vi "AnalogTriggers.vi"(1 "Limits":T5, 2 "Sources":T4, 3 "DutyCycles":T1, 4 "AnalogInputs":u16[](array[numeric])=[0, 0, 0, 0, 0, 0, 0, 0]) -> (0 "Outputs":T2)   [LabVIEW 2019]
uses:
  Controls/AnalogTrigger_Limits.ctl
  Controls/AnalogTrigger_Sources.ctl
  Controls/AnalogTrigger_Outputs.ctl
  Helpers/AnalogTriggerOutput.ctl
  Controls/DutyCycle_Outputs.ctl
  <vilib>/rvi/Emulation/niFpgaSctlEmulationGetInTimedLoop.vi
  <vilib>/rvi/Emulation/niFpgaProcessEmulError.vi
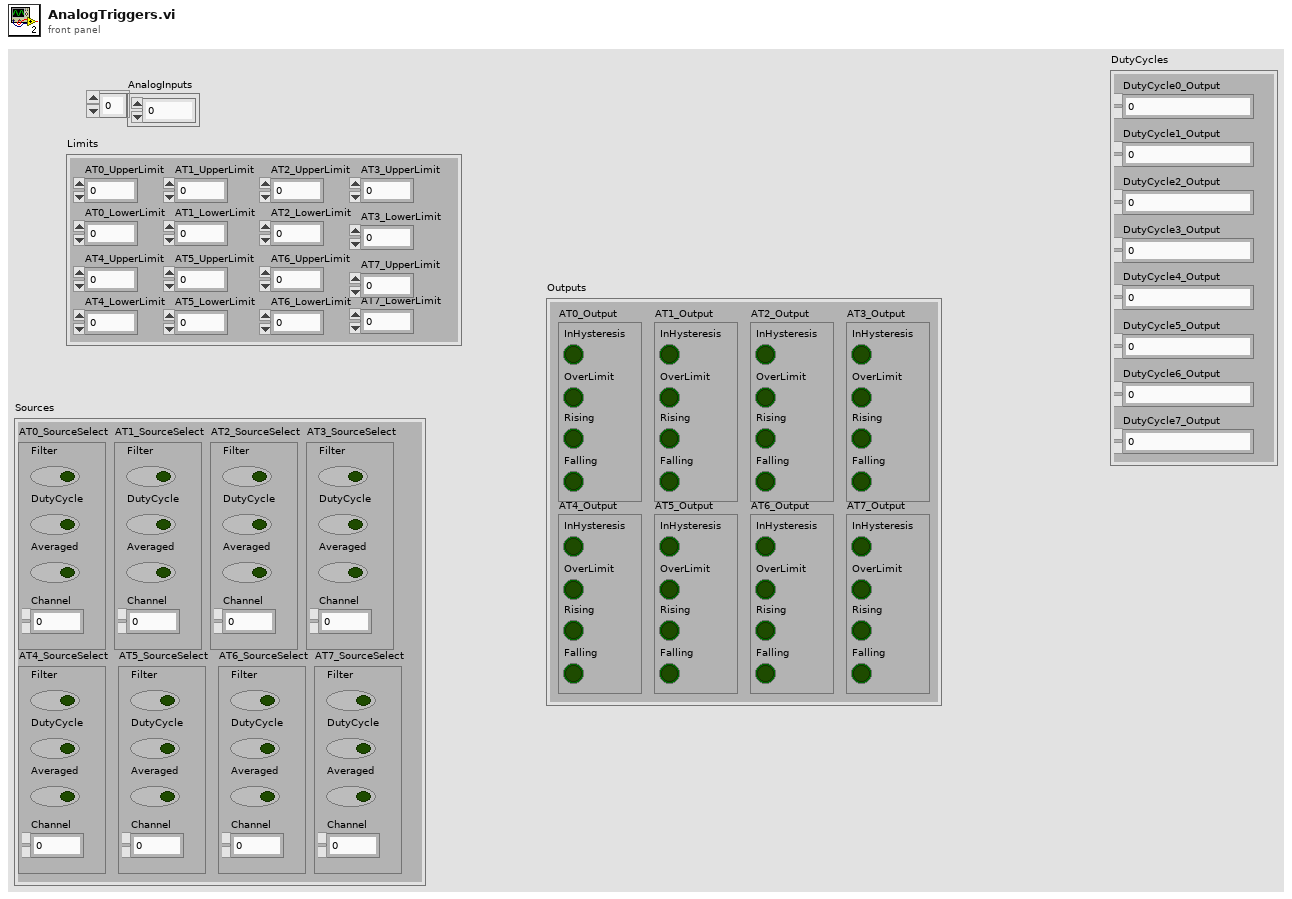
[diagram p1: front panel]
types:
  T1 = typedef "DutyCycle_Outputs.ctl" = cluster{"DutyCycle0_Output":fxp<+,31,31>, "DutyCycle1_Output":fxp<+,31,31>, "DutyCycle2_Output":fxp<+,31,31>, "DutyCycle3_Output":fxp<+,31,31>, "DutyCycle4_Output":fxp<+,31,31>, "DutyCycle5_Output":fxp<+,31,31>, "DutyCycle6_Output":fxp<+,31,31>, "DutyCycle7_Output":fxp<+,31,31>}
  T2 = typedef "AnalogTrigger_Outputs.ctl" = cluster{"AT0_Output":T3, "AT1_Output":T3, "AT2_Output":T3, "AT3_Output":T3, "AT4_Output":T3, "AT5_Output":T3, "AT6_Output":T3, "AT7_Output":T3}
  T3 = typedef "AnalogTriggerOutput.ctl" = cluster{"InHysteresis":bool, "OverLimit":bool, "Rising":bool, "Falling":bool}
  T4 = typedef "AnalogTrigger_Sources.ctl" = cluster{"AT0_SourceSelect":cluster{"Filter":bool, "DutyCycle":bool, "Averaged":bool, "Channel":fxp<+,3,3>}, "AT1_SourceSelect":cluster{"Filter":bool, "DutyCycle":bool, "Averaged":bool, "Channel":fxp<+,3,3>}, "AT2_SourceSelect":cluster{"Filter":bool, "DutyCycle":bool, "Averaged":bool, "Channel":fxp<+,3,3>}, "AT3_SourceSelect":cluster{"Filter":bool, "DutyCycle":bool, "Averaged":bool, "Channel":fxp<+,3,3>}, "AT4_SourceSelect":cluster{"Filter":bool, "DutyCycle":bool, "Averaged":bool, "Channel":fxp<+,3,3>}, "AT5_SourceSelect":cluster{"Filter":bool, "DutyCycle":bool, "Averaged":bool, "Channel":fxp<+,3,3>}, "AT6_SourceSelect":cluster{"Filter":bool, "DutyCycle":bool, "Averaged":bool, "Channel":fxp<+,3,3>}, "AT7_SourceSelect":cluster{"Filter":bool, "DutyCycle":bool, "Averaged":bool, "Channel":fxp<+,3,3>}}
  T5 = typedef "AnalogTrigger_Limits.ctl" = cluster{"AT0_LowerLimit":u32, "AT0_UpperLimit":u32, "AT1_LowerLimit":u32, "AT1_UpperLimit":u32, "AT2_LowerLimit":u32, "AT2_UpperLimit":u32, "AT3_LowerLimit":u32, "AT3_UpperLimit":u32, "AT4_LowerLimit":u32, "AT4_UpperLimit":u32, "AT5_LowerLimit":u32, "AT5_UpperLimit":u32, "AT6_LowerLimit":u32, "AT6_UpperLimit":u32, "AT7_LowerLimit":u32, "AT7_UpperLimit":u32}
  T6 = cluster{"Filter":bool, "DutyCycle":bool, "Averaged":bool, "Channel":fxp<+,3,3>}
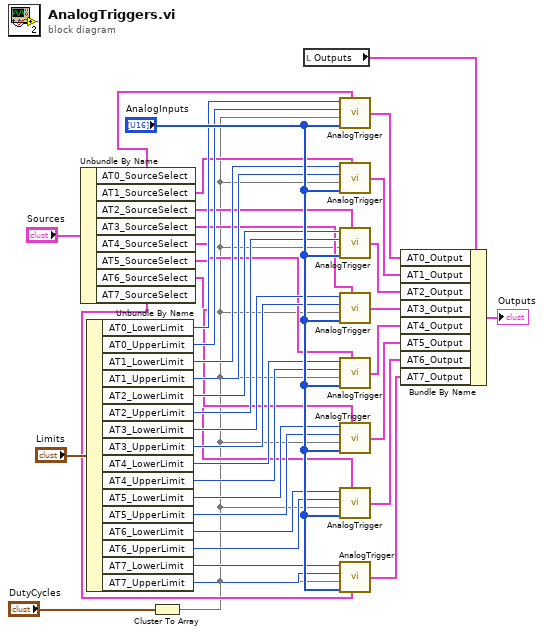
[diagram p0: block diagram]
diagram:
  n1 = Unbundle By Name("Sources") -> ("AT0_SourceSelect"=w20:T6, "AT1_SourceSelect"=w19:T6, "AT2_SourceSelect"=w18:T6, "AT3_SourceSelect"=w17:T6, "AT4_SourceSelect"=w16:T6, "AT5_SourceSelect"=w15:T6, "AT6_SourceSelect"=w14:T6, "AT7_SourceSelect"=w13:T6)
  n2 = Unbundle By Name("Limits") -> ("AT0_LowerLimit"=w37:u32, "AT0_UpperLimit"=w36:u32, "AT1_LowerLimit"=w35:u32, "AT1_UpperLimit"=w34:u32, "AT2_LowerLimit"=w33:u32, "AT2_UpperLimit"=w32:u32, "AT3_LowerLimit"=w31:u32, "AT3_UpperLimit"=w30:u32, "AT4_LowerLimit"=w29:u32, "AT4_UpperLimit"=w28:u32, "AT5_LowerLimit"=w27:u32, "AT5_UpperLimit"=w26:u32, "AT6_LowerLimit"=w25:u32, "AT6_UpperLimit"=w24:u32, "AT7_LowerLimit"=w23:u32, "AT7_UpperLimit"=w22:u32)
  n3 = Cluster To Array(cluster="DutyCycles") -> (array=w11:fxp<+,31,31>[])
  n4 = local read "Outputs"() -> (w10:T2)
  n5 = call "AnalogTrigger.vi"("LowerLimit"=w37, "UpperLimit"=w36, "DutyCycles"=w11, "AnalogInputs"="AnalogInputs", "SourceSelect"=w20) -> ("Output"=w8:T3)
  n6 = call "AnalogTrigger.vi"("LowerLimit"=w35, "UpperLimit"=w34, "DutyCycles"=w11, "AnalogInputs"="AnalogInputs", "SourceSelect"=w19) -> ("Output"=w7:T3)
  n7 = call "AnalogTrigger.vi"("LowerLimit"=w33, "UpperLimit"=w32, "DutyCycles"=w11, "AnalogInputs"="AnalogInputs", "SourceSelect"=w18) -> ("Output"=w6:T3)
  n8 = call "AnalogTrigger.vi"("LowerLimit"=w31, "UpperLimit"=w30, "DutyCycles"=w11, "AnalogInputs"="AnalogInputs", "SourceSelect"=w17) -> ("Output"=w5:T3)
  n9 = call "AnalogTrigger.vi"("LowerLimit"=w29, "UpperLimit"=w28, "DutyCycles"=w11, "AnalogInputs"="AnalogInputs", "SourceSelect"=w16) -> ("Output"=w4:T3)
  n10 = call "AnalogTrigger.vi"("LowerLimit"=w27, "UpperLimit"=w26, "DutyCycles"=w11, "AnalogInputs"="AnalogInputs", "SourceSelect"=w15) -> ("Output"=w3:T3)
  n11 = call "AnalogTrigger.vi"("LowerLimit"=w25, "UpperLimit"=w24, "DutyCycles"=w11, "AnalogInputs"="AnalogInputs", "SourceSelect"=w14) -> ("Output"=w2:T3)
  n12 = call "AnalogTrigger.vi"("LowerLimit"=w23, "UpperLimit"=w22, "DutyCycles"=w11, "AnalogInputs"="AnalogInputs", "SourceSelect"=w13) -> ("Output"=w1:T3)
  n13 = Bundle By Name(cluster=w10, "AT0_Output"=w8, "AT1_Output"=w7, "AT2_Output"=w6, "AT3_Output"=w5, "AT4_Output"=w4, "AT5_Output"=w3, "AT6_Output"=w2, "AT7_Output"=w1) -> (→"Outputs":T2)
